vi "集成干预测试数据存储.vi"(8 "error in (no error)":errorcluster, 11 "存储变量":T1={"时间标识"=timestamp(0 s since 1904-01-01), "参数"="", "数据类型"="N", "集成干预测试浓度值"=0.0, "集成干预前测试时间"=timestamp(0 s since 1904-01-01), "集成干预前测试浓度值"=0.0}) -> (0 "error out":errorcluster)   [LabVIEW 2016, in "PLC.lvlib"]
uses:
  PLC.lvlib
  <vilib>/addons/database/Auxilliary.llb/DB Tools Column Info.ctl
  <vilib>/addons/database/Auxilliary.llb/DB Tools DataTypes.ctl
  <vilib>/addons/database/NI_Database_API.lvlib
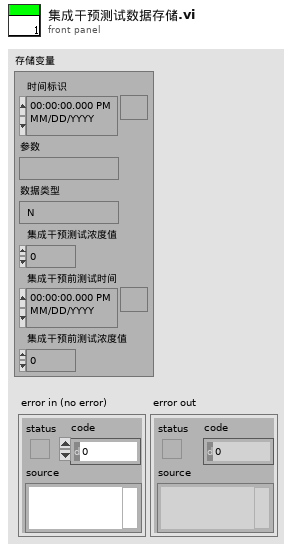
[diagram p1: front panel]
types:
  T1 = cluster{"时间标识":timestamp, "参数":string, "数据类型":string, "集成干预测试浓度值":dbl, "集成干预前测试时间":timestamp, "集成干预前测试浓度值":dbl}
  T2 = typedef "NI_Database_API.lvlib/DB Tools Column Info.ctl" = cluster{"column name":string, "data type":T3, "size":i32, "allow null?":bool}
  T3 = typedef "NI_Database_API.lvlib/DB Tools DataTypes.ctl" = enum16{"String", "Long (I32)", "Single (SGL)", "Double (DBL)", "Date/Time", "Binary"}
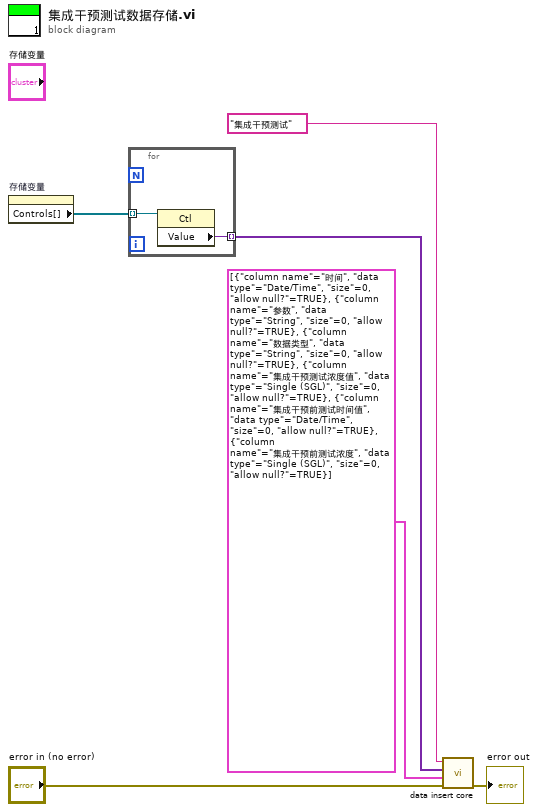
[diagram p0: block diagram]
diagram:
  n1 = property on="存储变量" class="Clust (严格)"() -> ("Controls[]"=w4:refnum<vi>[])  [unwired: 2 in, 2 out]
  n2 = for {
    tunnel: w4 -> [w8] mode=indexing
    tunnel: [w7] -> w3 mode=indexing
    n3 = property class="Ctl"(reference=w8) -> ("Value"=w7:variant)  [unwired: 1 in, 2 out]
  }
  n4 = call "data insert core.vi"("error in (no error)"="error in (no error)", "column information"=T2[] [{"column name"="时间", "data type"=enum."Date/Time", "size"=0, "allow null?"=TRUE}, {"column name"="参数", "data type"=enum."String", "size"=0, "allow null?"=TRUE}, {"column name"="数据类型", "data type"=enum."String", "size"=0, "allow null?"=TRUE}, {"column name"="集成干预测试浓度值", "data type"=enum."Single (SGL)", "size"=0, "allow null?"=TRUE}, {"column name"="集成干预前测试时间值", "data type"=enum."Date/Time", "size"=0, "allow null?"=TRUE}, {"column name"="集成干预前测试浓度", "data type"=enum."Single (SGL)", "size"=0, "allow null?"=TRUE}], "data"=w3, "table"="集成干预测试") -> ("error out"=→"error out":errorcluster)  [unwired: 7 in]
